vi "loadSettings.vi"(8 "error in (no error)":errorcluster, 9 "lookUpElementEvent":refnum<user-event>, 10 "whichSettings":string, 11 "TabCtl Refnum in":refnum<vi>) -> (0 "error out":errorcluster, 3 "TabCtl Refnum out":refnum<vi>)   [LabVIEW 2011, in "Views.lvlib" / "Camera.lvlib" / "andorSettingsViewer.lvclass"]
uses:
  andorSettingsViewer.lvclass
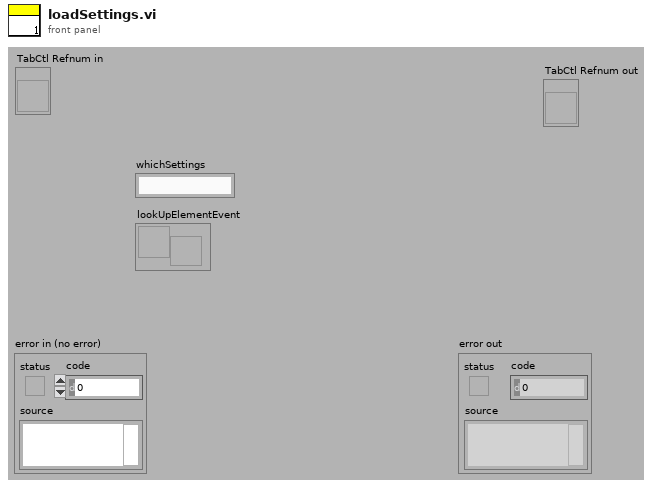
[diagram p1: front panel]
types:
  T1 = enum16{"Number", "String", "NumberArray", "StringArray"}
  T2 = cluster{"Label.Text":string, "whichSettings":string, "typeEnum":enum16{"Number", "String", "NumberArray", "StringArray"}}
  T3 = cluster{string, "whichSettings":string, "typeEnum":enum16{"Number", "String", "NumberArray", "StringArray"}}
  T4 = cluster{string, string, "typeEnum":enum16{"Number", "String", "NumberArray", "StringArray"}}
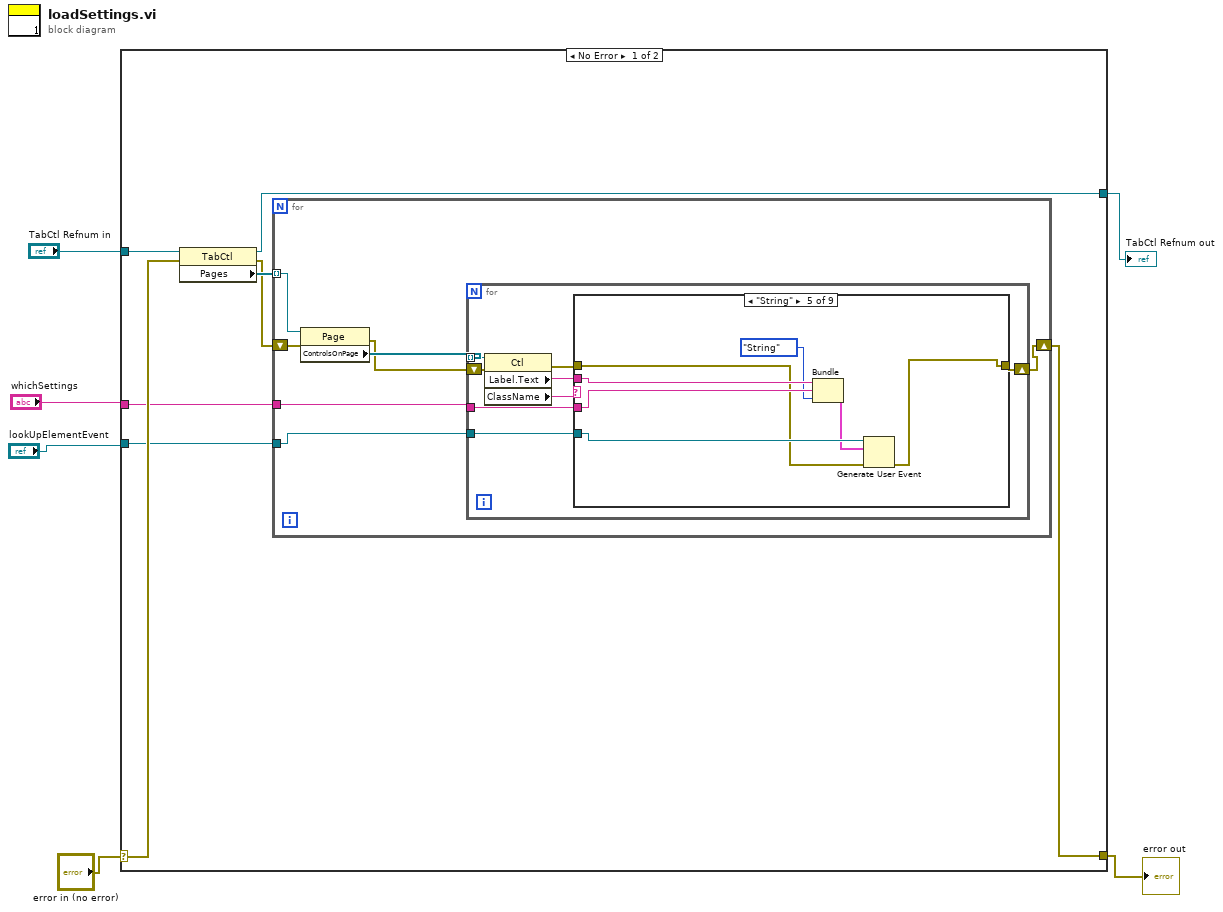
[diagram p0: block diagram]
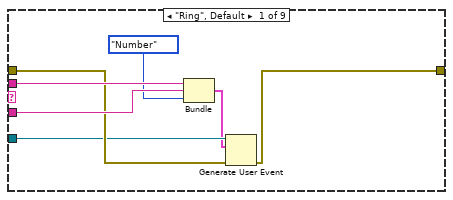
[diagram p2: hidden frame]
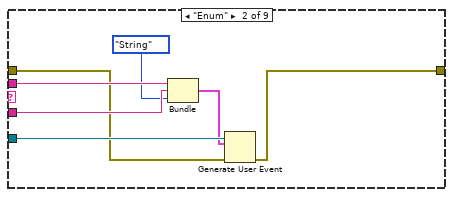
[diagram p3: hidden frame]
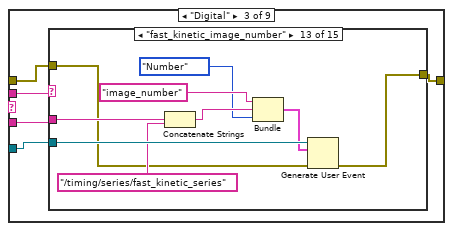
[diagram p4: hidden frame]
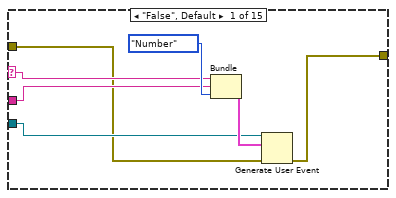
[diagram p5: hidden frame]
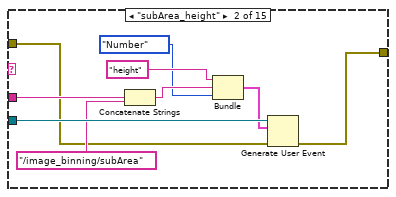
[diagram p6: hidden frame]
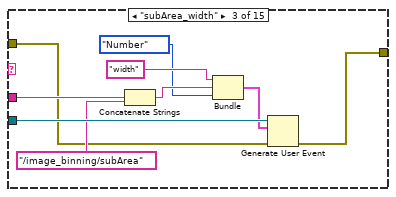
[diagram p7: hidden frame]
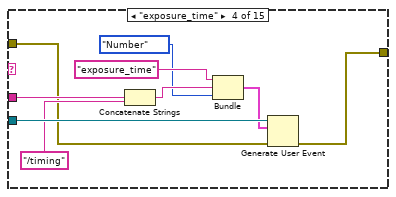
[diagram p8: hidden frame]
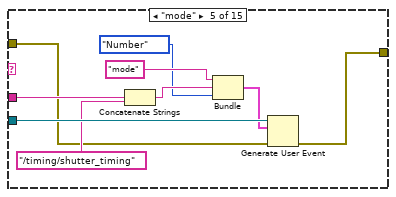
[diagram p9: hidden frame]
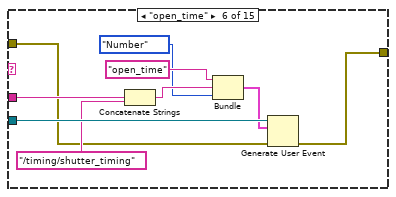
[diagram p10: hidden frame]
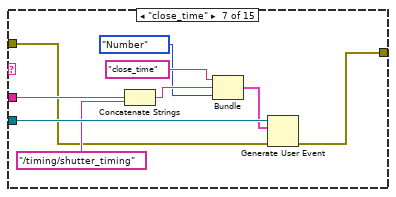
[diagram p11: hidden frame]
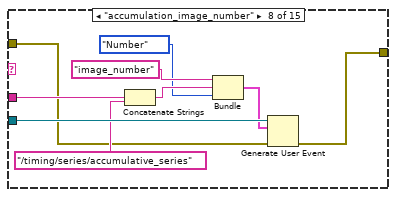
[diagram p12: hidden frame]
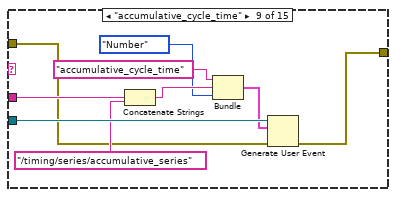
[diagram p13: hidden frame]
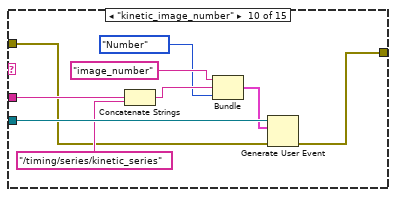
[diagram p14: hidden frame]
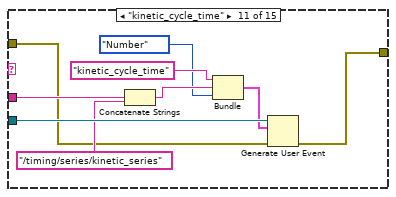
[diagram p15: hidden frame]
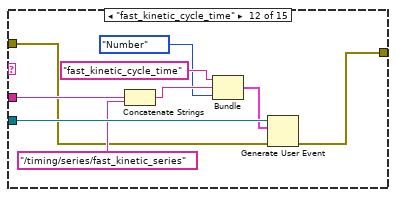
[diagram p16: hidden frame]
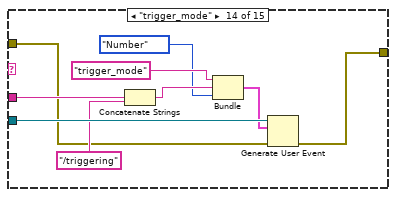
[diagram p17: hidden frame]
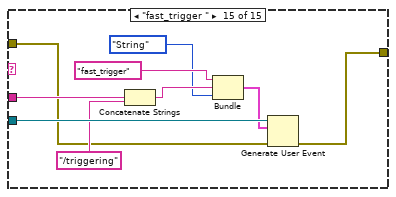
[diagram p18: hidden frame]
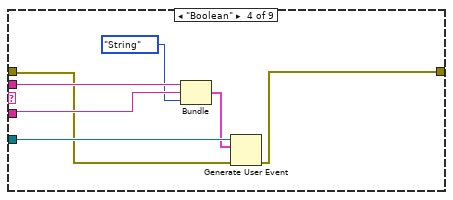
[diagram p19: hidden frame]
diagram:
  n1 = case shown="No Error" "error in (no error)" {
    selector: "error in (no error)" -> [w12 w228]
    tunnel: [w9 w228] -> w5
    tunnel: "whichSettings" -> [w11 _]
    tunnel: "lookUpElementEvent" -> [w10 _]
    tunnel: "TabCtl Refnum in" -> [w8 w227]
    tunnel: [w7 w227] -> w2
    frame No Error {
      n2 = property class="TabCtl"(reference=w8, error in=w12) -> (reference out=w7:refnum<vi>, error out=w13:errorcluster, "Pages"=w14:refnum<vi>[])
      n3 = for {
        shift-right: [w20] -> w9
        shift-left: w13 -> [w21]
        tunnel: w11 -> [w18]
        tunnel: w14 -> [w16] mode=indexing
        tunnel: w10 -> [w15]
        n4 = property class="Page"(reference=w16, error in=w21) -> (error out=w17:errorcluster, "ControlsOnPage"=w19:refnum<vi>[])  [unwired: 1 out]
        n5 = for {
          tunnel: w19 -> [w29] mode=indexing
          shift-right: [w25] -> w20
          shift-left: w17 -> [w28]
          tunnel: w15 -> [w23]
          tunnel: w18 -> [w24]
          n6 = property class="Ctl"(reference=w29, error in=w28) -> (error out=w26:errorcluster, "Label.Text"=w22:string, "ClassName"=w27:string)  [unwired: 1 out]
          n7 = case shown="\"String\"" w27 {
            tunnel: w26 -> [w33 w38 w44 w182 w189 w196 w197 w198 w200]
            tunnel: w22 -> [w36 w43 w45 w188 w195 _ _ _ w201]
            tunnel: [w31 w37 w48 w183 w192 w196 w197 w198 w199] -> w25
            tunnel: w24 -> [w35 w42 w46 w187 w194 _ _ _ w202]
            tunnel: w23 -> [w32 w40 w47 w185 w193 _ _ _ w203]
            frame "Ring", Default {
              n8 = Bundle("Label.Text"=w36, "whichSettings"=w35, "typeEnum"=T1."Number") -> (w30:T2)  [unwired: 1 in]
              n9 = Generate User Event(user event=w32, event data cluster=w30, error in=w33) -> (error out=w31:errorcluster)  [unwired: 1 out]
            }
            frame "Enum" {
              n10 = Bundle("Label.Text"=w43, "whichSettings"=w42, "typeEnum"=T1."String") -> (w39:T2)  [unwired: 1 in]
              n11 = Generate User Event(user event=w40, event data cluster=w39, error in=w38) -> (error out=w37:errorcluster)  [unwired: 1 out]
            }
            frame "Digital" {
              n12 = case shown="\"fast_kinetic_image_number\"" w45 {
                selector: w45 -> [w51 _ _ _ _ _ _ _ _ _ _ _ _ _ _]
                tunnel: w47 -> [w52 w64 w73 w82 w91 w100 w109 w118 w127 w136 w145 w154 w163 w172 w181]
                tunnel: [w53 w57 w66 w75 w84 w93 w102 w111 w120 w129 w138 w147 w156 w165 w174] -> w48
                tunnel: w46 -> [w50 w63 w72 w81 w90 w99 w108 w117 w126 w135 w144 w153 w162 w171 w180]
                tunnel: w44 -> [w49 w56 w65 w74 w83 w92 w101 w110 w119 w128 w137 w146 w155 w164 w173]
                frame "False", Default {
                  n13 = Bundle(w51, "whichSettings"=w50, "typeEnum"=T1."Number") -> (w54:T3)  [unwired: 1 in]
                  n14 = Generate User Event(user event=w52, event data cluster=w54, error in=w49) -> (error out=w53:errorcluster)  [unwired: 1 out]
                }
                frame "subArea_height" {
                  n15 = Concatenate Strings(w63, "/image_binning/subArea") -> (w60:string)
                  n16 = Bundle("height", w60, "typeEnum"=T1."Number") -> (w58:T4)  [unwired: 1 in]
                  n17 = Generate User Event(user event=w64, event data cluster=w58, error in=w56) -> (error out=w57:errorcluster)  [unwired: 1 out]
                }
                frame "subArea_width" {
                  n18 = Concatenate Strings(w72, "/image_binning/subArea") -> (w69:string)
                  n19 = Bundle("width", w69, "typeEnum"=T1."Number") -> (w67:T4)  [unwired: 1 in]
                  n20 = Generate User Event(user event=w73, event data cluster=w67, error in=w65) -> (error out=w66:errorcluster)  [unwired: 1 out]
                }
                frame "exposure_time" {
                  n21 = Concatenate Strings(w81, "/timing") -> (w78:string)
                  n22 = Bundle("exposure_time", w78, "typeEnum"=T1."Number") -> (w76:T4)  [unwired: 1 in]
                  n23 = Generate User Event(user event=w82, event data cluster=w76, error in=w74) -> (error out=w75:errorcluster)  [unwired: 1 out]
                }
                frame "mode" {
                  n24 = Concatenate Strings(w90, "/timing/shutter_timing") -> (w87:string)
                  n25 = Bundle("mode", w87, "typeEnum"=T1."Number") -> (w85:T4)  [unwired: 1 in]
                  n26 = Generate User Event(user event=w91, event data cluster=w85, error in=w83) -> (error out=w84:errorcluster)  [unwired: 1 out]
                }
                frame "open_time" {
                  n27 = Concatenate Strings(w99, "/timing/shutter_timing") -> (w96:string)
                  n28 = Bundle("open_time", w96, "typeEnum"=T1."Number") -> (w94:T4)  [unwired: 1 in]
                  n29 = Generate User Event(user event=w100, event data cluster=w94, error in=w92) -> (error out=w93:errorcluster)  [unwired: 1 out]
                }
                frame "close_time" {
                  n30 = Concatenate Strings(w108, "/timing/shutter_timing") -> (w105:string)
                  n31 = Bundle("close_time", w105, "typeEnum"=T1."Number") -> (w103:T4)  [unwired: 1 in]
                  n32 = Generate User Event(user event=w109, event data cluster=w103, error in=w101) -> (error out=w102:errorcluster)  [unwired: 1 out]
                }
                frame "accumulation_image_number" {
                  n33 = Concatenate Strings(w117, "/timing/series/accumulative_series") -> (w114:string)
                  n34 = Bundle("image_number", w114, "typeEnum"=T1."Number") -> (w112:T4)  [unwired: 1 in]
                  n35 = Generate User Event(user event=w118, event data cluster=w112, error in=w110) -> (error out=w111:errorcluster)  [unwired: 1 out]
                }
                frame "accumulative_cycle_time" {
                  n36 = Concatenate Strings(w126, "/timing/series/accumulative_series") -> (w123:string)
                  n37 = Bundle("accumulative_cycle_time", w123, "typeEnum"=T1."Number") -> (w121:T4)  [unwired: 1 in]
                  n38 = Generate User Event(user event=w127, event data cluster=w121, error in=w119) -> (error out=w120:errorcluster)  [unwired: 1 out]
                }
                frame "kinetic_image_number" {
                  n39 = Concatenate Strings(w135, "/timing/series/kinetic_series") -> (w132:string)
                  n40 = Bundle("image_number", w132, "typeEnum"=T1."Number") -> (w130:T4)  [unwired: 1 in]
                  n41 = Generate User Event(user event=w136, event data cluster=w130, error in=w128) -> (error out=w129:errorcluster)  [unwired: 1 out]
                }
                frame "kinetic_cycle_time" {
                  n42 = Concatenate Strings(w144, "/timing/series/kinetic_series") -> (w141:string)
                  n43 = Bundle("kinetic_cycle_time", w141, "typeEnum"=T1."Number") -> (w139:T4)  [unwired: 1 in]
                  n44 = Generate User Event(user event=w145, event data cluster=w139, error in=w137) -> (error out=w138:errorcluster)  [unwired: 1 out]
                }
                frame "fast_kinetic_cycle_time" {
                  n45 = Concatenate Strings(w153, "/timing/series/fast_kinetic_series") -> (w150:string)
                  n46 = Bundle("fast_kinetic_cycle_time", w150, "typeEnum"=T1."Number") -> (w148:T4)  [unwired: 1 in]
                  n47 = Generate User Event(user event=w154, event data cluster=w148, error in=w146) -> (error out=w147:errorcluster)  [unwired: 1 out]
                }
                frame "fast_kinetic_image_number" {
                  n48 = Concatenate Strings(w162, "/timing/series/fast_kinetic_series") -> (w159:string)
                  n49 = Bundle("image_number", w159, "typeEnum"=T1."Number") -> (w157:T4)  [unwired: 1 in]
                  n50 = Generate User Event(user event=w163, event data cluster=w157, error in=w155) -> (error out=w156:errorcluster)  [unwired: 1 out]
                }
                frame "trigger_mode" {
                  n51 = Concatenate Strings(w171, "/triggering") -> (w168:string)
                  n52 = Bundle("trigger_mode", w168, "typeEnum"=T1."Number") -> (w166:T4)  [unwired: 1 in]
                  n53 = Generate User Event(user event=w172, event data cluster=w166, error in=w164) -> (error out=w165:errorcluster)  [unwired: 1 out]
                }
                frame "fast_trigger " {
                  n54 = Concatenate Strings(w180, "/triggering") -> (w177:string)
                  n55 = Bundle("fast_trigger", w177, "typeEnum"=T1."String") -> (w175:T4)  [unwired: 1 in]
                  n56 = Generate User Event(user event=w181, event data cluster=w175, error in=w173) -> (error out=w174:errorcluster)  [unwired: 1 out]
                }
              }
            }
            frame "Boolean" {
              n57 = Bundle("Label.Text"=w188, "whichSettings"=w187, "typeEnum"=T1."String") -> (w184:T2)  [unwired: 1 in]
              n58 = Generate User Event(user event=w185, event data cluster=w184, error in=w182) -> (error out=w183:errorcluster)  [unwired: 1 out]
            }
            frame "String" {
              n59 = Bundle("Label.Text"=w195, "whichSettings"=w194, "typeEnum"=T1."String") -> (w190:T2)  [unwired: 1 in]
              n60 = Generate User Event(user event=w193, event data cluster=w190, error in=w189) -> (error out=w192:errorcluster)  [unwired: 1 out]
            }
            frame "Path" {
            }
            frame "Cluster" {
            }
            frame "Array" {
            }
            frame "MulticolumnListbox" {
              n61 = case shown="\"track_positions\"" w201 {
                tunnel: w203 -> [_ w217 w226]
                tunnel: w200 -> [w204 w205 w218]
                tunnel: [w204 w209 w219] -> w199
                tunnel: w202 -> [_ w208 w225]
                frame "False", Default {
                }
                frame "track_positions" {
                  w213 = T1."StringArray" ("typeEnum")
                  n62 = Concatenate Strings(w208, "/image_binning/track_positions") -> (w206:string)
                  n63 = Bundle("top", w206, "typeEnum"=w213) -> (w215:T4)  [unwired: 1 in]
                  n64 = Generate User Event(user event=w217, event data cluster=w215, error in=w205) -> (user event out=w211:refnum<user-event>, error out=w210:errorcluster)
                  n65 = Bundle("bottom", w206, "typeEnum"=w213) -> (w214:T4)  [unwired: 1 in]
                  n66 = Generate User Event(user event=w211, event data cluster=w214, error in=w210) -> (error out=w209:errorcluster)  [unwired: 1 out]
                }
                frame "subArea_coordinate" {
                  n67 = Concatenate Strings(w225, "/image_binning/subArea") -> (w222:string)
                  n68 = Bundle("coordinate", w222, "typeEnum"=T1."StringArray") -> (w220:T4)  [unwired: 1 in]
                  n69 = Generate User Event(user event=w226, event data cluster=w220, error in=w218) -> (error out=w219:errorcluster)  [unwired: 1 out]
                }
              }
            }
          }
        }
      }
    }
    frame Error {
    }
  }
  "error out" <- w5
  "TabCtl Refnum out" <- w2
